vi "OE1022D_DATA Transmit.vi"(0 "Input Data":u8[](array[numeric])) -> (1 "CH A_Parameter Values":T2, 2 "CH B_Parameter Values":T2, 3 "Total Date Array":dbl[][](array[numeric]), 4 "PLL&Overload":T1)   [LabVIEW 2019]
panel:
  out "B_XitaD2":dbl[](array[numeric])
  out "B_RD2":dbl[](array[numeric])
  out "B_XitaD1":dbl[](array[numeric])
  out "B_RD1":dbl[](array[numeric])
  out "B_Xita":dbl[](array[numeric])
  out "B_R":dbl[](array[numeric])
  out "B_YD2":dbl[](array[numeric])
  out "B_XD2":dbl[](array[numeric])
  out "B_YD1":dbl[](array[numeric])
  out "B_XD1":dbl[](array[numeric])
  out "B_Noise":dbl[](array[numeric])
  out "B_Frequency":dbl[](array[numeric])
  out "B_Y":dbl[](array[numeric])
  out "B_X":dbl[](array[numeric])
  out "A_X":dbl[](array[numeric])
  out "A_Y":dbl[](array[numeric])
  out "A_Frequency":dbl[](array[numeric])
  out "A_Noise":dbl[](array[numeric])
  out "A_XD1":dbl[](array[numeric])
  out "A_YD1":dbl[](array[numeric])
  out "A_XD2":dbl[](array[numeric])
  out "A_YD2":dbl[](array[numeric])
  out "AUXADC1":dbl[](array[numeric])
  out "AUXADC2":dbl[](array[numeric])
  out "AUXADC3":dbl[](array[numeric])
  out "AUXADC4":dbl[](array[numeric])
  out "A_R":dbl[](array[numeric])
  out "A_Xita":dbl[](array[numeric])
  out "A_RD1":dbl[](array[numeric])
  out "A_XitaD1":dbl[](array[numeric])
  out "A_RD2":dbl[](array[numeric])
  out "A_XitaD2":dbl[](array[numeric])
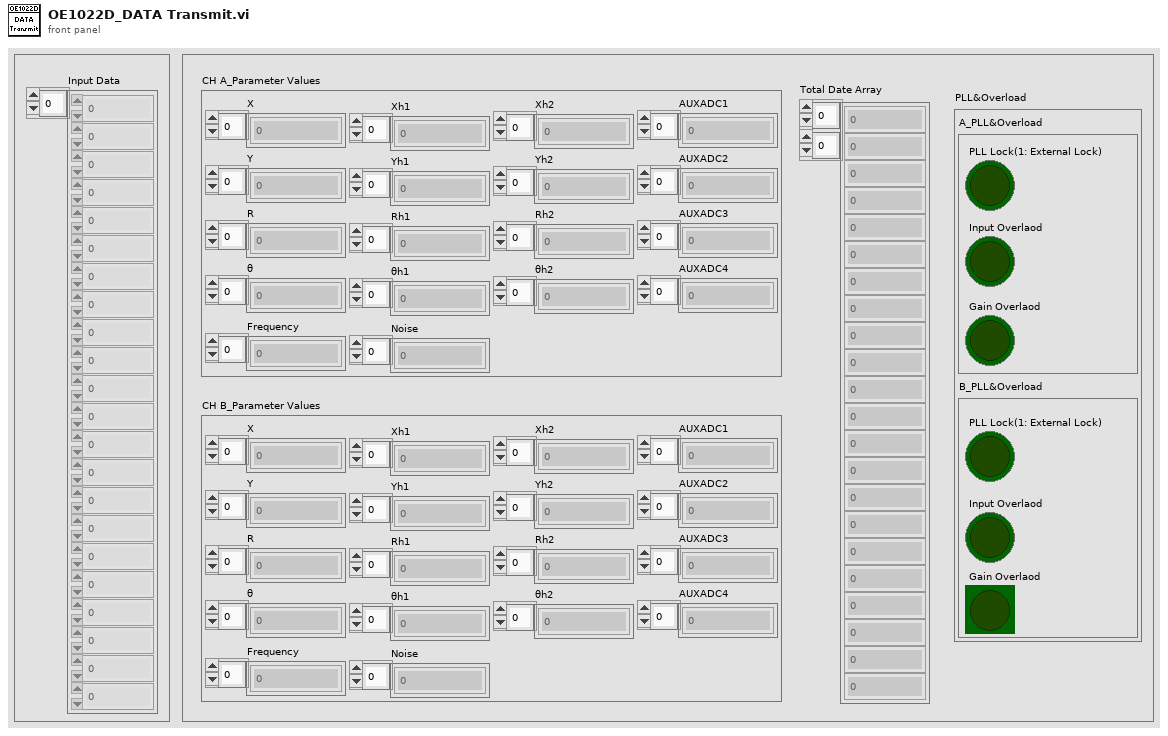
[diagram p1: front panel]
types:
  T1 = cluster{"A_PLL&Overload":cluster{"PLL Lock(1: External Lock)":bool, "Input Overlaod":bool, "Gain Overlaod":bool}, "B_PLL&Overload":cluster{"PLL Lock(1: External Lock)":bool, "Input Overlaod":bool, "Gain Overlaod":bool}}
  T2 = cluster{"X":dbl[], "Y":dbl[], "R":dbl[], "θ":dbl[], "Noise":dbl[], "Frequency":dbl[], "Xh1":dbl[], "Yh1":dbl[], "Rh1":dbl[], "θh1":dbl[], "Xh2":dbl[], "Yh2":dbl[], "Rh2":dbl[], "θh2":dbl[], "AUXADC1":dbl[], "AUXADC2":dbl[], "AUXADC3":dbl[], "AUXADC4":dbl[]}
  T3 = cluster{cluster{bool, bool, bool}, cluster{bool, bool, bool}}
  T4 = cluster{"A_X":dbl[], "A_Y":dbl[], "A_R":dbl[], "A_Xita":dbl[], "A_Noise":dbl[], "A_Frequency":dbl[], "A_XD1":dbl[], "A_YD1":dbl[], "A_RD1":dbl[], "A_XitaD1":dbl[], "A_XD2":dbl[], "A_YD2":dbl[], "A_RD2":dbl[], "A_XitaD2":dbl[], "AUXADC1":dbl[], "AUXADC2":dbl[], "AUXADC3":dbl[], "AUXADC4":dbl[]}
  T5 = cluster{"B_X":dbl[], "B_Y":dbl[], "B_R":dbl[], "B_Xita":dbl[], "B_Noise":dbl[], "B_Frequency":dbl[], "B_XD1":dbl[], "B_YD1":dbl[], "B_RD1":dbl[], "B_XitaD1":dbl[], "B_XD2":dbl[], "B_YD2":dbl[], "B_RD2":dbl[], "B_XitaD2":dbl[], "AUXADC1":dbl[], "AUXADC2":dbl[], "AUXADC3":dbl[], "AUXADC4":dbl[]}
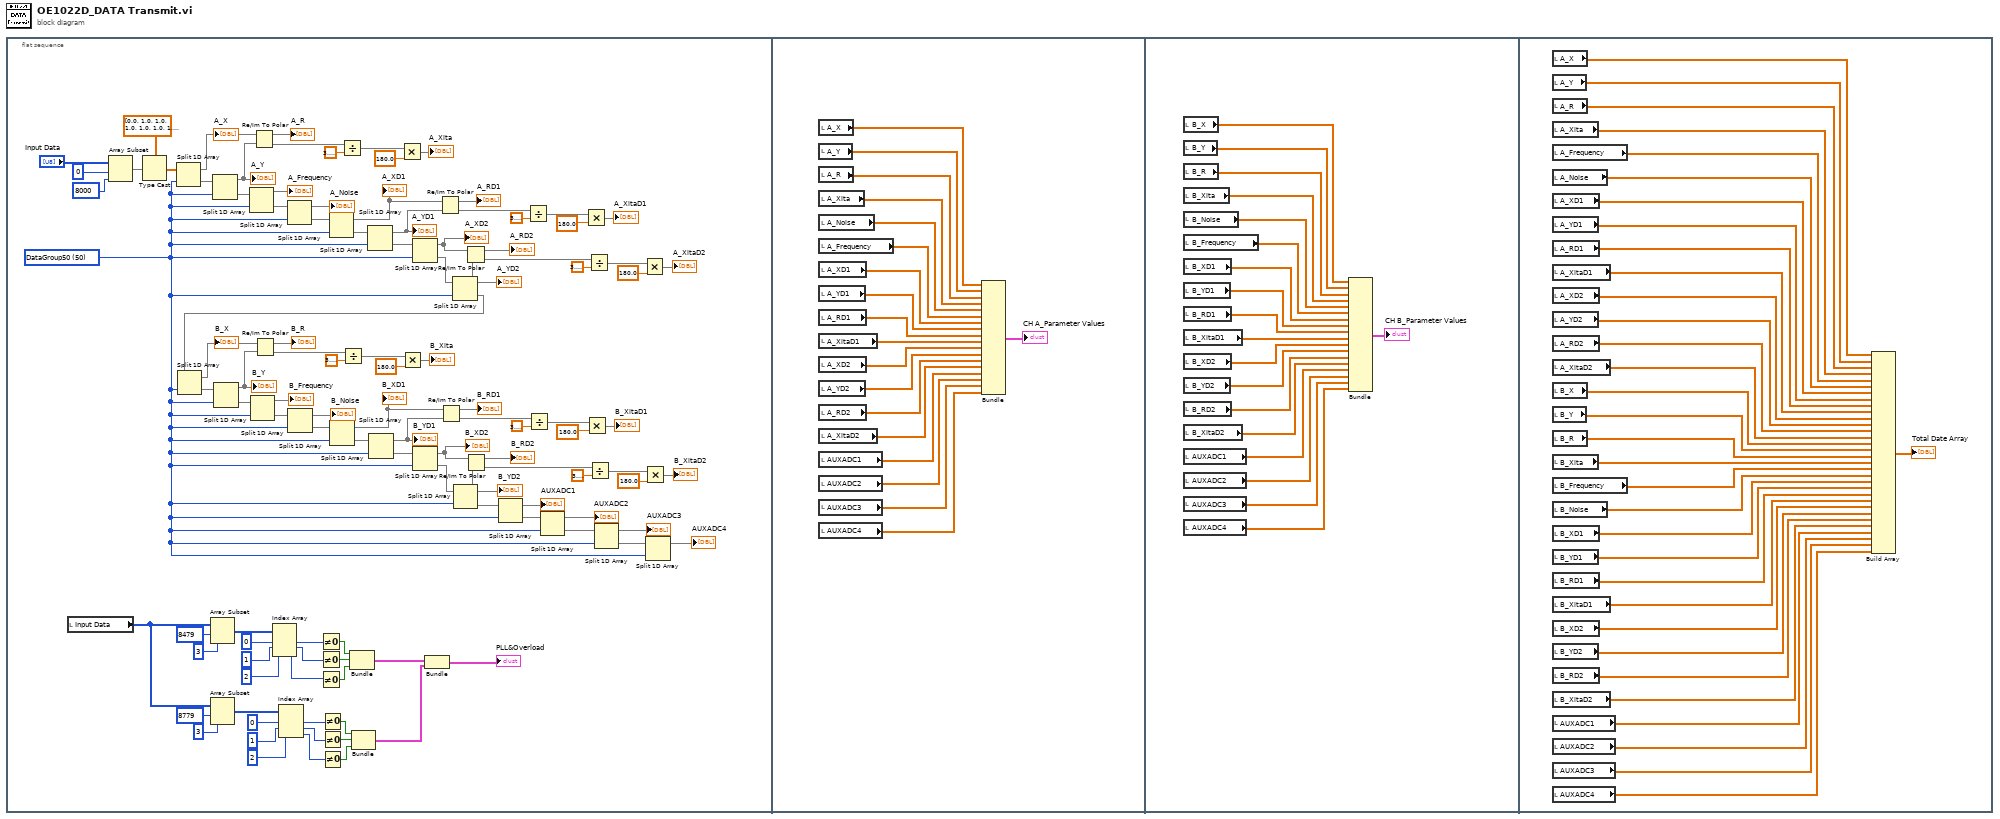
[diagram p0: block diagram]
diagram:
  n1 = flat-sequence {
    frame #0 {
      w34 = u16 50 items=["unsignedInt8"=1, "unsignedInt16"=2, "unsignedInt32"=4, "unsignedInt64"=8, "Float"=80, "Double"=160, "StartLength"=2240, "DataGroup50"=50, "DataGroup100"=100, "DataGroup20"=20] ("数据类型")
      n2 = local read "Input Data"() -> (w24:u8[])
      n3 = Array Subset(array="Input Data", index=0 ("索引"), length=8000 ("长度")) -> (w107:u8[])
      n4 = Type Cast(type=dbl[] [0.0, 1.0, 1.0, 1.0, 1.0, 1.0, 1.0, 1.0, 1.0, 1.0, 1.0, 1.0, 1.0, 1.0, 1.0, 1.0, 1.0, 1.0, 1.0, 1.0, 1.0, 1.0, 1.0, 1.0, 1.0, 1.0, 1.0, 1.0, 1.0, 1.0, 1.0, 1.0, 1.0, 1.0, 1.0, 1.0, 1.0, 1.0, 1.0, 1.0, 1.0, 1.0, 1.0, 1.0, 1.0, 1.0, 1.0, 1.0, 1.0, 1.0, 1.0, 1.0, 1.0, 1.0, 1.0, 1.0, 1.0, 1.0, 1.0, 1.0, 1.0, 1.0, 1.0, 1.0, 1.0, 1.0, 1.0, 1.0, 1.0, 1.0, 1.0, 1.0, 1.0, 1.0, 1.0, 1.0, 1.0, 1.0, 1.0, 1.0, 1.0, 1.0, 1.0, 1.0, 1.0, 1.0, 1.0, 1.0, 1.0, 1.0, 1.0, 1.0, 1.0, 1.0, 1.0, 1.0, 1.0, 1.0, 1.0, 1.0, 1.0, 1.0, 1.0, 1.0, 1.0, 1.0, 1.0, 1.0, 1.0, 1.0, 1.0, 1.0, 1.0, 1.0, 1.0, 1.0, 1.0, 1.0, 1.0, 1.0, 1.0, 1.0, 1.0, 1.0, 1.0, 1.0, 1.0, 1.0, 1.0, 1.0, 1.0, 1.0, 1.0, 1.0, 1.0, 1.0, 1.0, 1.0, 1.0, 1.0, 1.0, 1.0, 1.0, 1.0, 1.0, 1.0, 1.0, 1.0, 1.0, 1.0, 1.0, 1.0, 1.0, 1.0, 1.0, 1.0, 1.0, 1.0, 1.0, 1.0, 1.0, 1.0, 1.0, 1.0, 1.0, 1.0, 1.0, 1.0, 1.0, 1.0, 1.0, 1.0, 1.0, 1.0, 1.0, 1.0, 1.0, 1.0, 1.0, 1.0, 1.0, 1.0, 1.0, 1.0, 1.0, 1.0, 1.0, 1.0, 1.0, 1.0, 1.0, 1.0, 1.0, 1.0, 1.0, 1.0, 1.0, 1.0, 1.0, 1.0, 1.0, 1.0, 1.0, 1.0, 1.0, 1.0, 1.0, 1.0, 1.0, 1.0, 1.0, 1.0, 1.0, 1.0, 1.0, 1.0, 1.0, 1.0, 1.0, 1.0, 1.0, 1.0, 1.0, 1.0, 1.0, 1.0, 1.0, 1.0, 1.0, 1.0, 1.0, 1.0, 1.0, 1.0, 1.0, 1.0, 1.0, 1.0, 1.0, 1.0, 1.0, 1.0, 1.0, 1.0, 1.0, 1.0, 1.0, 1.0, 1.0, 1.0, 1.0, 1.0, 1.0, 1.0, 1.0, 1.0, 1.0, 1.0, 1.0, 1.0, 1.0, 1.0, 1.0, 1.0, 1.0, 1.0, 1.0, 1.0, 1.0, 1.0, 1.0, 1.0, 1.0, 1.0, 1.0, 1.0, 1.0, 1.0, 1.0, 1.0, 1.0, 1.0, 1.0, 1.0, 1.0, 1.0, 1.0, 1.0, 1.0, 1.0, 1.0, 1.0, 1.0, 1.0, 1.0, 1.0, 1.0, 1.0, 1.0, 1.0, 1.0, 1.0, 1.0, 1.0, 1.0, 1.0, 1.0, 1.0, 1.0, 1.0, 1.0, 1.0, 1.0, 1.0, 1.0, 1.0, 1.0, 1.0, 1.0, 1.0, 1.0, 1.0, 1.0, 1.0, 1.0, 1.0, 1.0, 1.0, 1.0, 1.0, 1.0, 1.0, 1.0, 1.0, 1.0, 1.0, 1.0, 1.0, 1.0, 1.0, 1.0, 1.0, 1.0, 1.0, 1.0, 1.0, 1.0, 1.0, 1.0, 1.0, 1.0, 1.0, 1.0, 1.0, 1.0, 1.0, 1.0, 1.0, 1.0, 1.0, 1.0, 1.0, 1.0, 1.0, 1.0, 1.0, 1.0, 1.0, 1.0, 1.0, 1.0, 1.0, 1.0, 1.0, 1.0, 1.0, 1.0, 1.0, 1.0, 1.0, 1.0, 1.0, 1.0, 1.0, 1.0, 1.0, 1.0, 1.0, 1.0, 1.0, 1.0, 1.0, 1.0, 1.0, 1.0, 1.0, 1.0, 1.0, 1.0, 1.0, 0.0, 1.0, 1.0, 1.0, 1.0, 1.0, 1.0, 1.0, 1.0, 1.0, 1.0, 1.0, 1.0, 1.0, 1.0, 1.0, 1.0, 1.0, 1.0, 1.0, 1.0, 1.0, 1.0, 1.0, 1.0, 1.0, 1.0, 1.0, 1.0, 1.0, 1.0, 1.0, 1.0, 1.0, 1.0, 1.0, 1.0, 1.0, 1.0, 1.0, 1.0, 1.0, 1.0, 1.0, 1.0, 1.0, 1.0, 1.0, 1.0, 1.0, 1.0, 1.0, 1.0, 1.0, 1.0, 1.0, 1.0, 1.0, 1.0, 1.0, 1.0, 1.0, 1.0, 1.0, 1.0, 1.0, 1.0, 1.0, 1.0, 1.0, 1.0, 1.0, 1.0, 1.0, 1.0, 1.0, 1.0, 1.0, 1.0, 1.0, 1.0, 1.0, 1.0, 1.0, 1.0, 1.0, 1.0, 1.0, 1.0, 1.0, 1.0, 1.0, 1.0, 1.0, 1.0, 1.0, 1.0, 1.0, 1.0, 1.0, 1.0, 1.0, 1.0, 1.0, 1.0, 1.0, 1.0, 1.0, 1.0, 1.0, 1.0, 1.0, 1.0, 1.0, 1.0, 1.0, 1.0, 1.0, 1.0, 1.0, 1.0, 1.0, 1.0, 1.0, 1.0, 1.0, 1.0, 1.0, 1.0, 1.0, 1.0, 1.0, 1.0, 1.0, 1.0, 1.0, 1.0, 1.0, 1.0, 1.0, 1.0, 1.0, 1.0, 1.0, 1.0, 1.0, 1.0, 1.0, 1.0, 1.0, 1.0, 1.0, 1.0, 1.0, 1.0, 1.0, 1.0, 1.0, 1.0, 1.0, 1.0, 1.0, 1.0, 1.0, 1.0, 1.0, 1.0, 1.0, 1.0, 1.0, 1.0, 1.0, 1.0, 1.0, 1.0, 1.0, 1.0, 1.0, 1.0, 1.0, 1.0, 1.0, 1.0, 1.0, 1.0, 1.0, 1.0, 1.0, 1.0, 1.0, 1.0, 1.0, 1.0, 1.0, 1.0, 1.0, 1.0, 1.0, 1.0, 1.0, 1.0, 1.0, 1.0, 1.0, 1.0, 1.0, 1.0, 1.0, 1.0, 1.0, 1.0, 1.0, 1.0, 1.0, 1.0, 1.0, 1.0, 1.0, 1.0, 1.0, 1.0, 1.0, 1.0, 1.0, 1.0, 1.0, 1.0, 1.0, 1.0, 1.0, 1.0, 1.0, 1.0, 1.0, 1.0, 1.0, 1.0, 1.0, 1.0, 1.0, 1.0, 1.0, 1.0, 1.0, 1.0, 1.0, 1.0, 1.0, 1.0, 1.0, 1.0, 1.0, 1.0, 1.0, 1.0, 1.0, 1.0, 1.0, 1.0, 1.0, 1.0, 1.0, 1.0, 1.0, 1.0, 1.0, 1.0, 1.0, 1.0, 1.0, 1.0, 1.0, 1.0, 1.0, 1.0, 1.0, 1.0, 1.0, 1.0, 1.0, 1.0, 1.0, 1.0, 1.0, 1.0, 1.0, 1.0, 1.0, 1.0, 1.0, 1.0, 1.0, 1.0, 1.0, 1.0, 1.0, 1.0, 1.0, 1.0, 1.0, 1.0, 1.0, 1.0, 1.0, 1.0, 1.0, 1.0, 1.0, 1.0, 1.0, 1.0, 1.0, 1.0, 1.0, 1.0, 1.0, 1.0, 1.0, 1.0, 1.0, 1.0, 1.0, 1.0, 1.0, 1.0, 1.0, 1.0, 1.0, 1.0, 1.0, 1.0, 1.0, 1.0, 1.0, 1.0, 1.0, 1.0, 1.0, 1.0, 1.0, 1.0, 1.0, 1.0, 1.0, 1.0, 1.0, 1.0, 1.0, 1.0, 1.0, 1.0, 1.0, 1.0, 1.0, 1.0, 1.0, 1.0, 1.0, 1.0, 1.0, 1.0, 1.0, 1.0, 1.0, 1.0, 1.0, 1.0, 1.0, 1.0, 1.0, 1.0, 1.0, 1.0, 1.0, 1.0, 1.0, 1.0, 1.0, 1.0, 1.0, 1.0, 1.0, 1.0, 1.0, 1.0, 1.0, 1.0, 1.0, 1.0, 1.0, 1.0, 1.0, 1.0, 1.0, 1.0, 1.0, 1.0, 1.0, 1.0, 1.0], x=w107) -> (*(type *) &x=w99:dbl[])
      n5 = Split 1D Array(array=w99, index=w34) -> (first subarray=w90:dbl[], second subarray=w100:dbl[])
      "A_X" <- w90
      n6 = Array Subset(array=w24, index=8479 ("索引"), length=3 ("长度")) -> (w16:u8[])
      n7 = Array Subset(array=w24, index=8779 ("索引"), length=3 ("长度")) -> (w9:u8[])
      n8 = Split 1D Array(array=w100, index=w34) -> (first subarray=w89:dbl[], second subarray=w108:dbl[])
      "A_Y" <- w89
      n9 = Split 1D Array(array=w108, index=w34) -> (first subarray=→"A_Frequency":dbl[], second subarray=w95:dbl[])
      n10 = Re/Im To Polar(2:w89, 3:w90) -> (0:w88:dbl[], 1:→"A_R":dbl[])
      n11 = Index Array(array=w16, index #1=0 ("索引"), index #2=1 ("索引"), index #3=2 ("索引")) -> (element #1=w8:u8, element #2=w7:u8, element #3=w6:u8)
      n12 = Index Array(array=w9, index #1=0 ("索引"), index #2=1 ("索引"), index #3=2 ("索引")) -> (element #1=w5:u8, element #2=w4:u8, element #3=w3:u8)
      n13 = Split 1D Array(array=w95, index=w34) -> (first subarray=→"A_Noise":dbl[], second subarray=w69:dbl[])
      n14 = Not Equal To 0?(x=w8) -> (x != 0?=w22:bool)
      n15 = Not Equal To 0?(x=w7) -> (x != 0?=w23:bool)
      n16 = Not Equal To 0?(x=w6) -> (x != 0?=w21:bool)
      n17 = Not Equal To 0?(x=w5) -> (x != 0?=w18:bool)
      n18 = Not Equal To 0?(x=w4) -> (x != 0?=w17:bool)
      n19 = Not Equal To 0?(x=w3) -> (x != 0?=w19:bool)
      n20 = Split 1D Array(array=w69, index=w34) -> (first subarray=w73:dbl[], second subarray=w103:dbl[])
      "A_XD1" <- w73
      n21 = Divide(x=w88, y=3.141592653589793) -> (x/y=w92:dbl[])
      n22 = Bundle(w22, w23, w21) -> (w20:cluster{bool, bool, bool})  [unwired: 1 in]
      n23 = Bundle(w18, w17, w19) -> (w2:cluster{bool, bool, bool})  [unwired: 1 in]
      n24 = Split 1D Array(array=w103, index=w34) -> (first subarray=w72:dbl[], second subarray=w109:dbl[])
      "A_YD1" <- w72
      n25 = Multiply(x=w92, y=180.0) -> (x*y=→"A_Xita":dbl[])
      n26 = Split 1D Array(array=w109, index=w34) -> (first subarray=w71:dbl[], second subarray=w110:dbl[])
      "A_XD2" <- w71
      n27 = Bundle(w20, w2) -> (→"PLL&Overload":T3)  [unwired: 1 in]
      n28 = Re/Im To Polar(2:w72, 3:w73) -> (0:w83:dbl[], 1:→"A_RD1":dbl[])
      n29 = Split 1D Array(array=w110, index=w34) -> (first subarray=w70:dbl[], second subarray=w33:dbl[])
      "A_YD2" <- w70
      n30 = Split 1D Array(array=w33, index=w34) -> (first subarray=w56:dbl[], second subarray=w61:dbl[])
      "B_X" <- w56
      n31 = Split 1D Array(array=w61, index=w34) -> (first subarray=w55:dbl[], second subarray=w65:dbl[])
      "B_Y" <- w55
      n32 = Split 1D Array(array=w65, index=w34) -> (first subarray=→"B_Frequency":dbl[], second subarray=w60:dbl[])
      n33 = Re/Im To Polar(2:w55, 3:w56) -> (0:w54:dbl[], 1:→"B_R":dbl[])
      n34 = Split 1D Array(array=w60, index=w34) -> (first subarray=→"B_Noise":dbl[], second subarray=w35:dbl[])
      n35 = Split 1D Array(array=w35, index=w34) -> (first subarray=w39:dbl[], second subarray=w64:dbl[])
      "B_XD1" <- w39
      n36 = Divide(x=w54, y=3.141592653589793) -> (x/y=w58:dbl[])
      n37 = Split 1D Array(array=w64, index=w34) -> (first subarray=w38:dbl[], second subarray=w66:dbl[])
      "B_YD1" <- w38
      n38 = Multiply(x=w58, y=180.0) -> (x*y=→"B_Xita":dbl[])
      n39 = Split 1D Array(array=w66, index=w34) -> (first subarray=w37:dbl[], second subarray=w67:dbl[])
      "B_XD2" <- w37
      n40 = Re/Im To Polar(2:w38, 3:w39) -> (0:w49:dbl[], 1:→"B_RD1":dbl[])
      n41 = Split 1D Array(array=w67, index=w34) -> (first subarray=w36:dbl[], second subarray=w32:dbl[])
      "B_YD2" <- w36
      n42 = Re/Im To Polar(2:w70, 3:w71) -> (0:w76:dbl[], 1:→"A_RD2":dbl[])
      n43 = Re/Im To Polar(2:w36, 3:w37) -> (0:w42:dbl[], 1:→"B_RD2":dbl[])
      n44 = Split 1D Array(array=w32, index=w34) -> (first subarray=→"AUXADC1":dbl[], second subarray=w104:dbl[])
      n45 = Divide(x=w83, y=3.141592653589793) -> (x/y=w81:dbl[])
      n46 = Divide(x=w49, y=3.141592653589793) -> (x/y=w47:dbl[])
      n47 = Split 1D Array(array=w104, index=w34) -> (first subarray=→"AUXADC2":dbl[], second subarray=w106:dbl[])
      n48 = Multiply(x=w81, y=180.0) -> (x*y=→"A_XitaD1":dbl[])
      n49 = Multiply(x=w47, y=180.0) -> (x*y=→"B_XitaD1":dbl[])
      n50 = Divide(x=w76, y=3.141592653589793) -> (x/y=w78:dbl[])
      n51 = Divide(x=w42, y=3.141592653589793) -> (x/y=w44:dbl[])
      n52 = Split 1D Array(array=w106, index=w34) -> (first subarray=→"AUXADC3":dbl[], second subarray=w105:dbl[])
      n53 = Multiply(x=w78, y=180.0) -> (x*y=→"A_XitaD2":dbl[])
      n54 = Multiply(x=w44, y=180.0) -> (x*y=→"B_XitaD2":dbl[])
      n55 = Split 1D Array(array=w105, index=w34) -> (first subarray=→"AUXADC4":dbl[])  [unwired: 1 out]
    }
    frame #1 {
      n56 = local read "A_X"() -> (w129:dbl[])
      n57 = local read "A_Y"() -> (w128:dbl[])
      n58 = local read "A_R"() -> (w127:dbl[])
      n59 = local read "A_Xita"() -> (w126:dbl[])
      n60 = local read "A_Noise"() -> (w125:dbl[])
      n61 = local read "A_Frequency"() -> (w124:dbl[])
      n62 = local read "A_XD1"() -> (w120:dbl[])
      n63 = local read "A_YD1"() -> (w119:dbl[])
      n64 = local read "A_RD1"() -> (w118:dbl[])
      n65 = local read "A_XitaD1"() -> (w117:dbl[])
      n66 = local read "A_XD2"() -> (w116:dbl[])
      n67 = local read "A_YD2"() -> (w115:dbl[])
      n68 = local read "A_RD2"() -> (w114:dbl[])
      n69 = local read "A_XitaD2"() -> (w113:dbl[])
      n70 = local read "AUXADC1"() -> (w121:dbl[])
      n71 = local read "AUXADC2"() -> (w122:dbl[])
      n72 = local read "AUXADC3"() -> (w123:dbl[])
      n73 = local read "AUXADC4"() -> (w111:dbl[])
      n74 = Bundle("A_X"=w129, "A_Y"=w128, "A_R"=w127, "A_Xita"=w126, "A_Noise"=w125, "A_Frequency"=w124, "A_XD1"=w120, "A_YD1"=w119, "A_RD1"=w118, "A_XitaD1"=w117, "A_XD2"=w116, "A_YD2"=w115, "A_RD2"=w114, "A_XitaD2"=w113, "AUXADC1"=w121, "AUXADC2"=w122, "AUXADC3"=w123, "AUXADC4"=w111) -> (→"CH A_Parameter Values":T4)  [unwired: 1 in]
    }
    frame #2 {
      n75 = local read "B_X"() -> (w148:dbl[])
      n76 = local read "B_Y"() -> (w147:dbl[])
      n77 = local read "B_R"() -> (w146:dbl[])
      n78 = local read "B_Xita"() -> (w145:dbl[])
      n79 = local read "B_Noise"() -> (w144:dbl[])
      n80 = local read "B_Frequency"() -> (w143:dbl[])
      n81 = local read "B_XD1"() -> (w138:dbl[])
      n82 = local read "B_YD1"() -> (w137:dbl[])
      n83 = local read "B_RD1"() -> (w136:dbl[])
      n84 = local read "B_XitaD1"() -> (w135:dbl[])
      n85 = local read "B_XD2"() -> (w134:dbl[])
      n86 = local read "B_YD2"() -> (w133:dbl[])
      n87 = local read "B_RD2"() -> (w132:dbl[])
      n88 = local read "B_XitaD2"() -> (w131:dbl[])
      n89 = local read "AUXADC1"() -> (w139:dbl[])
      n90 = local read "AUXADC2"() -> (w140:dbl[])
      n91 = local read "AUXADC3"() -> (w141:dbl[])
      n92 = local read "AUXADC4"() -> (w142:dbl[])
      n93 = Bundle("B_X"=w148, "B_Y"=w147, "B_R"=w146, "B_Xita"=w145, "B_Noise"=w144, "B_Frequency"=w143, "B_XD1"=w138, "B_YD1"=w137, "B_RD1"=w136, "B_XitaD1"=w135, "B_XD2"=w134, "B_YD2"=w133, "B_RD2"=w132, "B_XitaD2"=w131, "AUXADC1"=w139, "AUXADC2"=w140, "AUXADC3"=w141, "AUXADC4"=w142) -> (→"CH B_Parameter Values":T5)  [unwired: 1 in]
    }
    frame #3 {
      n94 = local read "A_X"() -> (w170:dbl[])
      n95 = local read "A_Y"() -> (w171:dbl[])
      n96 = local read "A_R"() -> (w172:dbl[])
      n97 = local read "A_Xita"() -> (w173:dbl[])
      n98 = local read "A_Frequency"() -> (w152:dbl[])
      n99 = local read "A_Noise"() -> (w151:dbl[])
      n100 = local read "A_XD1"() -> (w174:dbl[])
      n101 = local read "A_YD1"() -> (w175:dbl[])
      n102 = local read "A_RD1"() -> (w176:dbl[])
      n103 = local read "A_XitaD1"() -> (w177:dbl[])
      n104 = local read "A_XD2"() -> (w178:dbl[])
      n105 = local read "A_YD2"() -> (w179:dbl[])
      n106 = local read "A_RD2"() -> (w180:dbl[])
      n107 = local read "A_XitaD2"() -> (w181:dbl[])
      n108 = local read "B_X"() -> (w168:dbl[])
      n109 = local read "B_Y"() -> (w167:dbl[])
      n110 = local read "B_R"() -> (w166:dbl[])
      n111 = local read "B_Xita"() -> (w165:dbl[])
      n112 = local read "B_Frequency"() -> (w149:dbl[])
      n113 = local read "B_Noise"() -> (w150:dbl[])
      n114 = local read "B_XD1"() -> (w164:dbl[])
      n115 = local read "B_YD1"() -> (w163:dbl[])
      n116 = local read "B_RD1"() -> (w162:dbl[])
      n117 = local read "B_XitaD1"() -> (w161:dbl[])
      n118 = local read "B_XD2"() -> (w160:dbl[])
      n119 = local read "B_YD2"() -> (w159:dbl[])
      n120 = local read "B_RD2"() -> (w158:dbl[])
      n121 = local read "B_XitaD2"() -> (w157:dbl[])
      n122 = local read "AUXADC1"() -> (w156:dbl[])
      n123 = local read "AUXADC2"() -> (w155:dbl[])
      n124 = local read "AUXADC3"() -> (w154:dbl[])
      n125 = local read "AUXADC4"() -> (w153:dbl[])
      n126 = Build Array(w170, w171, w172, w173, w152, w151, w174, w175, w176, w177, w178, w179, w180, w181, w168, w167, w166, w165, w149, w150, w164, w163, w162, w161, w160, w159, w158, w157, w156, w155, w154, w153) -> (→"Total Date Array":dbl[][])
    }
  }
